vi "WSVCAP SHL Host LL SPI_RFFE Build DUT Mask.vi"(0 "DUT":T1, 7 "All DUTs":bool) -> (4 "Socket Mask [U16]":u16=132 format="%04x", 6 "Socket Mask Array":bool[](array[boolean]), 8 "DUT Mask":bool[](array[boolean]))   [LabVIEW 2012]
uses:
  Type Defs/WSVCAP SHL DUT Number Enum.ctl
panel:
  # "SKT 01"
  # "SKT 02"
  # "SKT 03"
  # "SKT 04"
  # "SKT 05"
  # "SKT 06"
  # "SKT 07"
  # "SKT 08"
  # "SKT 09"
  # "SKT 10"
  # "SKT 11"
  # "SKT 12"
  # "SKT 13"
  # "SKT 14"
  # "SKT 15"
  # "SKT 16"
  # "DUT 01"
  # "DUT 02"
  # "DUT 03"
  # "DUT 04"
  # "DUT 05"
  # "DUT 06"
  # "DUT 07"
  # "DUT 08"
  # "DUT 09"
  # "DUT 10"
  # "DUT 11"
  # "DUT 12"
  # "DUT 13"
  # "DUT 14"
  # "DUT 15"
  # "DUT 16"
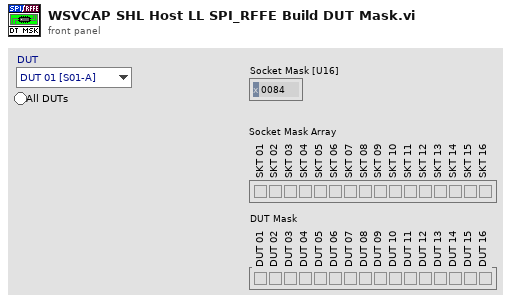
[diagram p1: front panel]
types:
  T1 = typedef "WSVCAP SHL DUT Number Enum.ctl" = enum16{"DUT 01 [S01-A]", "DUT 02 [S02-B]", "DUT 03 [S03-C]", "DUT 04 [S04-D]", "DUT 05 [S05-E]", "DUT 06 [S06-F]", "DUT 07 [S07-G]", "DUT 08 [S08-H]", "DUT 09 [S09-I]", "DUT 10 [S10-J]", "DUT 11 [S11-K]", "DUT 12 [S12-L]", "DUT 13 [S13-M]", "DUT 14 [S14-N]", "DUT 15 [S15-O]", "DUT 16 [S16-P]"}
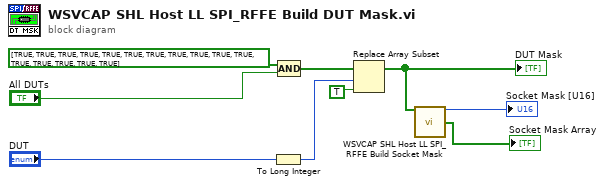
[diagram p0: block diagram]
diagram:
  n1 = To Long Integer(number="DUT") -> (32bit integer=w4:i32)
  n2 = Compound Arithmetic op=AND(bool[] [TRUE, TRUE, TRUE, TRUE, TRUE, TRUE, TRUE, TRUE, TRUE, TRUE, TRUE, TRUE, TRUE, TRUE, TRUE, TRUE], "All DUTs") -> (w7:bool[])
  n3 = Replace Array Subset(array=w7, new element=TRUE, index=w4) -> (w3:bool[])
  "DUT Mask" <- w3
  n4 = call "WSVCAP SHL Host LL SPI_RFFE Build Socket Mask.vi"("DUT Mask"=w3) -> ("Socket Mask [U16]"=→"Socket Mask [U16]":u16, "Socket Mask Array"=→"Socket Mask Array":bool[])  [unwired: 13 in]
